vi "ToString.vi"(8 "error in (no error)":errorcluster, 11 "U32 D Element in":refnum<class "String D Element.lvclass">) -> (0 "error out":errorcluster, 2 "String":string, 3 "U32 D Element out":refnum<class "String D Element.lvclass">)   [LabVIEW 2018, in "D Datagrid Library.lvlib" / "String D Element.lvclass"]
uses:
  String D Element.lvclass
  String D Element.lvclass/String D Element.ctl
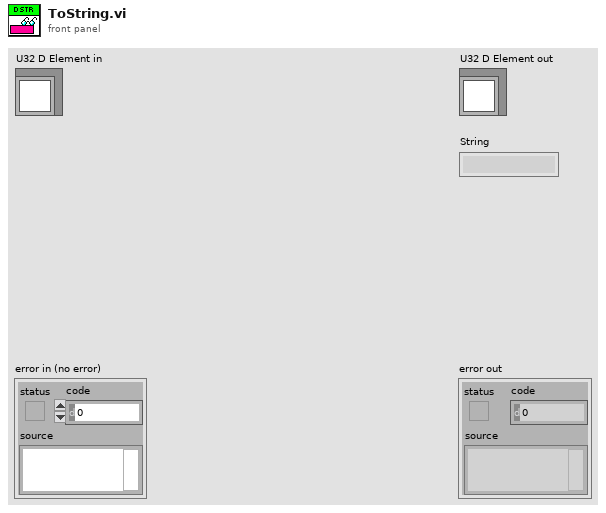
[diagram p1: front panel]
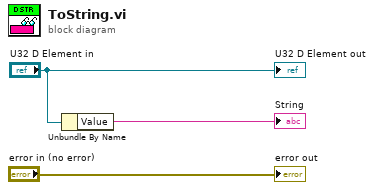
[diagram p0: block diagram]
diagram:
  n1 = Unbundle By Name("U32 D Element in") -> ("Value"=→"String":string)
  "error out" <- "error in (no error)"
  "U32 D Element out" <- "U32 D Element in"
